vi "ProdaNG.WabcoPart.Get.vi"(8 "error in (no error)":errorcluster, 9 "WabcoPartId (-1: use WabcoNumber)":i32=-1, 10 "WabcoNumber (\"\": use WabcoPartId)":string, 11 "dbHandleIn":i32) -> (0 "error out":errorcluster, 1 "ProductName":string, 2 "WabcoPart":T1, 3 "dbHandle":i32)   [LabVIEW 2016]
doc: "This function returns a product structure for a product, which is identified by a part and a serial number.\nImportant information: The field 'individual' was taken over from the field 'allgemein' of the legacy data directly. Because of this most products have the value 0 further on and only a few the value 1. \nParameter:\nhandle is an Integer, which is returned by the function Login() at the creation of a new connection.\nwabcoPartId is the Id of the part.\nserialNumber is the serial number of the product for the part above.\nproduct is a pointer on a product structure, which is filled if the returncode is 0. The structure must be defined in the calling program.\n\nReturncodes:\n0 No error\n< 0 ORACLE Error code\n6 (ERROR_INVALID_HANDLE) in case of an invalid handle\n1403 Record does not exist"
uses:
  Controls/ProdaNG.WabcoPart.ctl
  Controls/ProdaNG.WabcoPartSize.ctl
  prodllNG.dll
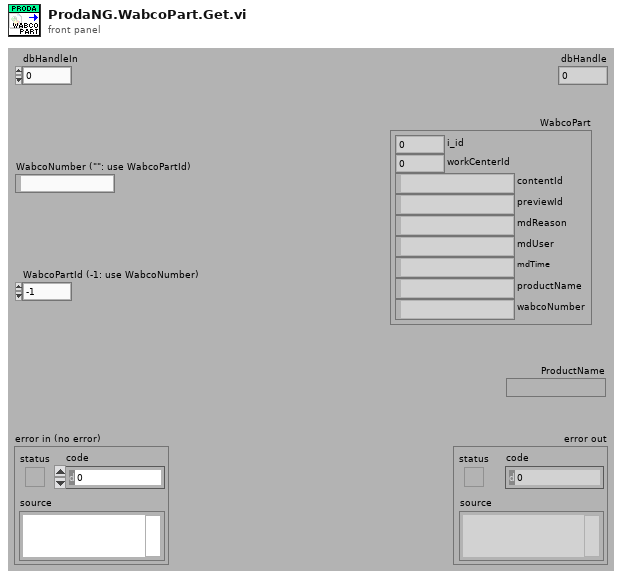
[diagram p1: front panel]
types:
  T1 = typedef "ProdaNG.WabcoPart.ctl" = cluster{"i_id":i32, "workCenterId":i32, "contentId":string, "previewId":string, "mdReason":string, "mdUser":string, "mdTime":string, "productName":string, "wabcoNumber":string}
  T2 = typedef "ProdaNG.WabcoPartSize.ctl" = cluster{"i_id":i32, "workCenterId":i32, "contentId":i32, "previewId":i32, "mdReason":i32, "mdUser":i32, "mdTime":i32, "productName":i32, "wabcoNumber":i32}
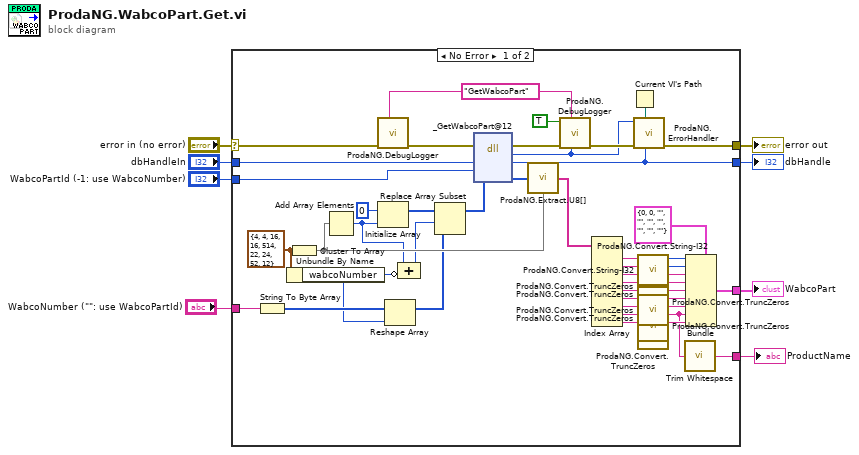
[diagram p0: block diagram]
diagram:
  n1 = case shown="No Error" "error in (no error)" {
    selector: "error in (no error)" -> [w49 w56]
    tunnel: [w54 w56] -> w7
    tunnel: "dbHandleIn" -> [w51 w55]
    tunnel: [w52 w55] -> w5
    tunnel: "WabcoPartId (-1: use WabcoNumber)" -> [w42 _]
    tunnel: [w22 _] -> w3
    tunnel: "WabcoNumber (\"\": use WabcoPartId)" -> [w20 _]
    tunnel: [w9 _] -> w1
    frame No Error {
      w17 = T2 {"i_id"=4, "workCenterId"=4, "contentId"=16, "previewId"=16, "mdReason"=514, "mdUser"=22, "mdTime"=24, "productName"=52, "wabcoNumber"=12} ("WabcoPart")
      w45 = "GetWabcoPart" ("cmd")
      n2 = String To Byte Array(string=w20) -> (unsigned byte array=w14:u8[])
      n3 = Unbundle By Name(w17) -> ("wabcoNumber"=w12:i32)
      n4 = Cluster To Array(cluster=w17) -> (array=w41:i32[])
      n5 = Add Array Elements(numeric array=w41) -> (sum=w16:i32)
      n6 = call "ProdaNG.DebugLogger.vi"("cmd"=w45, "error in (no error)"=w49) -> ("error out"=w48:errorcluster)  [unwired: 9 in]
      n7 = Initialize Array(u8 0 ("element"), w16) -> (w19:u8[])
      n8 = Reshape Array(w14, w12) -> (w13:u8[])
      n9 = Compound Arithmetic op=unknown(w16, invert w12) -> (w15:i32)
      n10 = Replace Array Subset(array=w19, new element=w13, index=w15) -> (w18:u8[])
      n11 = dll-call lib="D:/svn/LineTraceSystem/SOFTWARE/sources/Database/ProdaNG/prodllNG.dll" fn="_GetWabcoPart@12" ("ProDLL wrapper.dll:ProDLL_wrapper_GetWabcoParts_GetData")(error in=w48, "dbHandle"=w51, "wabcoPartId"=w42, "processStepPtr"=w18) -> (error out=w47:errorcluster, "return type"=w44:i32, "dbHandle"=w52:i32, "processStepPtr"=w40:u8[])  [unwired: 3 in, 1 out]
      n12 = call "ProdaNG.Extract.U8[].vi"("unsigned byte array"=w40, "Sizes"=w41) -> ("Elements"=w21:string[])
      n13 = call "ProdaNG.DebugLogger.vi"("return type"=w44, "cmd"=w45, "error in (no error)"=w47, "done? (F)"=TRUE) -> ("error out"=w46:errorcluster)  [unwired: 7 in]
      n14 = Index Array(array=w21) -> (element #1=w34:string, element #2=w33:string, element #3=w28:string, element #4=w29:string, element #5=w37:string, element #6=w39:string, element #7=w32:string, element #8=w31:string, element #9=w24:string)  [unwired: 9 in]
      n15 = Current VI's Path() -> (path=w53:path)
      n16 = call "ProdaNG.ErrorHandler.vi"("dbHandleIn"=w52, "Path"=w53, "error in"=w46, "output_parameter"=w44) -> ("error out"=w54:errorcluster)  [unwired: 7 in]
      n17 = call "ProdaNG.Convert.String-I32.vi"("unsigned byte string"=w34) -> ("32bit integer"=w23:i32)  [unwired: 10 in]
      n18 = call "ProdaNG.Convert.String-I32.vi"("unsigned byte string"=w33) -> ("32bit integer"=w35:i32)  [unwired: 10 in]
      n19 = call "ProdaNG.Convert.TruncZeros.vi"("string with \\0s"=w28) -> ("LV string"=w27:string)  [unwired: 10 in]
      n20 = call "ProdaNG.Convert.TruncZeros.vi"("string with \\0s"=w29) -> ("LV string"=w26:string)  [unwired: 10 in]
      n21 = call "ProdaNG.Convert.TruncZeros.vi"("string with \\0s"=w37) -> ("LV string"=w36:string)  [unwired: 10 in]
      n22 = call "ProdaNG.Convert.TruncZeros.vi"("string with \\0s"=w39) -> ("LV string"=w38:string)  [unwired: 10 in]
      n23 = call "ProdaNG.Convert.TruncZeros.vi"("string with \\0s"=w32) -> ("LV string"=w30:string)  [unwired: 10 in]
      n24 = call "ProdaNG.Convert.TruncZeros.vi"("string with \\0s"=w31) -> ("LV string"=w10:string)  [unwired: 10 in]
      n25 = call "ProdaNG.Convert.TruncZeros.vi"("string with \\0s"=w24) -> ("LV string"=w25:string)  [unwired: 10 in]
      n26 = call <vilib>:"Trim Whitespace.vi"("string"=w10) -> ("trimmed string"=w9:string)  [unwired: 1 in]
      n27 = Bundle(cluster=T1 {"i_id"=0, "workCenterId"=0, "contentId"="", "previewId"="", "mdReason"="", "mdUser"="", "mdTime"="", "productName"="", "wabcoNumber"=""} ("WabcoPart"), "i_id"=w23, "workCenterId"=w35, "contentId"=w27, "previewId"=w26, "mdReason"=w36, "mdUser"=w38, "mdTime"=w30, "productName"=w10, "wabcoNumber"=w25) -> (w22:T1)
    }
    frame Error {
    }
  }
  "error out" <- w7
  "dbHandle" <- w5
  "WabcoPart" <- w3
  "ProductName" <- w1
